vi "Add A File.vi"(5 "Size":u32, 7 "Parrent":string, 10 "Name":string, 11 "Map":T1) -> (3 "Map Out":T1)   [LabVIEW 2020]
uses:
  MAP_Structure.ctl
  Cluster_Item Data.ctl
  <vilib>/Utility/miscctls.llb/LVMapReplaceAction.ctl
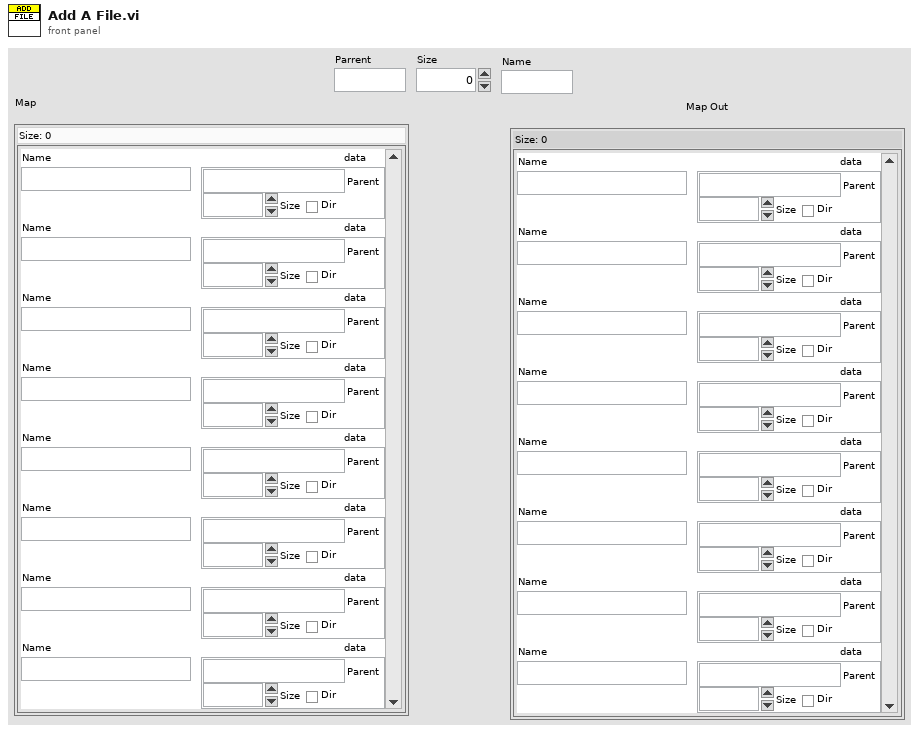
[diagram p1: front panel]
types:
  T1 = typedef "MAP_Structure.ctl" = map{string, T2}
  T2 = typedef "Cluster_Item Data.ctl" = cluster{"Parent":string, "Size":u32, "Dir":bool}
  T3 = typedef "LVMapReplaceAction.ctl" = enum32{"Modify Entry only if found", "Add or Modify Entry", "Delete Entry"}
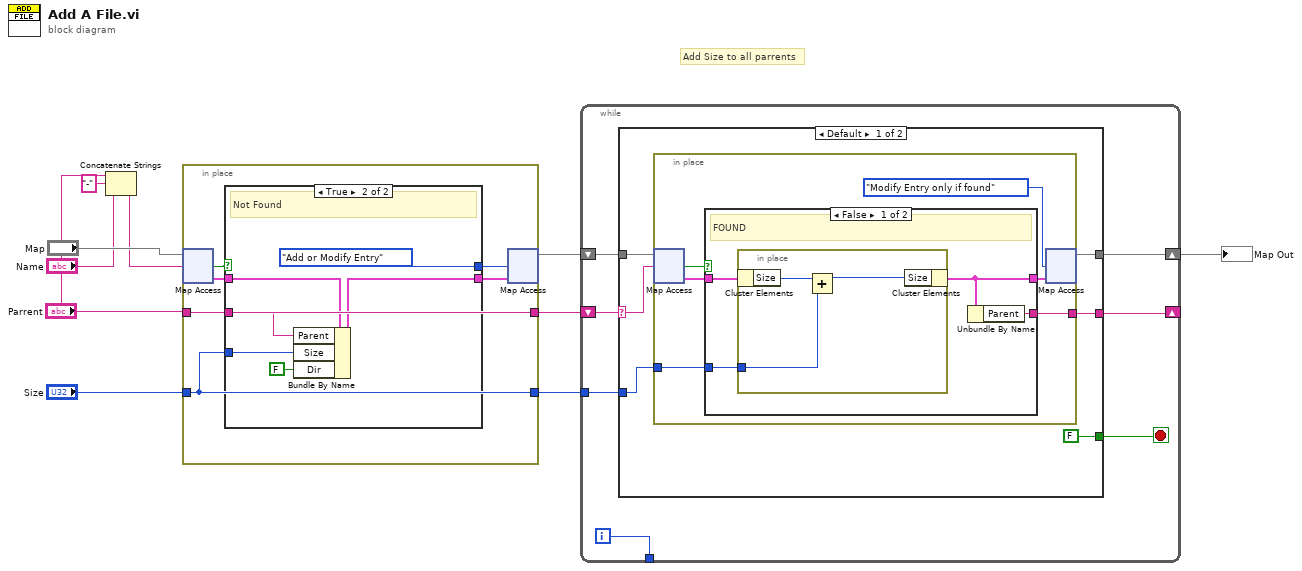
[diagram p0: block diagram]
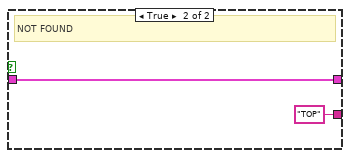
[diagram p2: hidden frame]
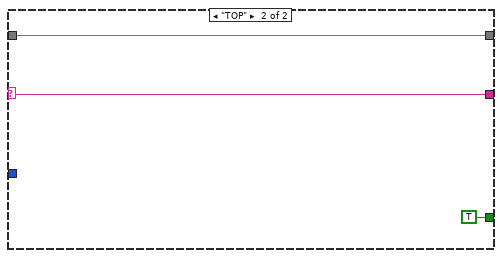
[diagram p3: hidden frame]
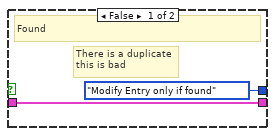
[diagram p4: hidden frame]
diagram:
  # "Add Size to all parrents"
  n1 = Concatenate Strings("Parrent", "-" ("string"), "Name") -> (w1:string)
  n2 = in-place {
    in-place-border: "Parrent" -> [w12]
    in-place-border: "Size" -> [w13]
    in-place-border: [w13] -> w6
    in-place-border: [w12] -> w5
    n3 = in-place-map #1("Map", w1) -> (w16:T2, w11:bool)  [unwired: 1 in]
    n4 = case shown="True" w11 {
      tunnel: w16 -> [w18 w24]
      tunnel: [w18 w23] -> w15
      tunnel: [LVMapReplaceAction."Modify Entry only if found" ("action") LVMapReplaceAction."Add or Modify Entry" ("action")] -> w14
      tunnel: w13 -> [_ w21]
      tunnel: w12 -> [_ w20]
      frame False {
        # "There is a duplicate\nthis is bad"
        # "Found"
      }
      frame True {
        # "Not Found"
        n5 = Bundle By Name(cluster=w24, "Parent"=w20, "Size"=w21, "Dir"=FALSE) -> (w23:T2)
      }
    }
    n6 = in-place-map #1(w15, w14) -> (w8:T1)  [unwired: 2 out]
  }
  n7 = while {
    shift-right: [w29] -> w7
    shift-left: w8 -> [w30]
    tunnel: w6 -> [w26]
    shift-right: [w27] -> _
    shift-left: w5 -> [w31]
    tunnel: [w25] -> _
    i -> [w25]
    stop <- w28 stop-if-true
    n8 = case shown="Default" w31 {
      selector: w31 -> [w34 w54]
      tunnel: w30 -> [w36 w55]
      tunnel: [w35 w55] -> w29
      tunnel: [FALSE TRUE] -> w28
      tunnel: [w33 w54] -> w27
      tunnel: w26 -> [w32 _]
      frame Default {
        n9 = in-place {
          in-place-border: [w41] -> w33
          in-place-border: w32 -> [w39]
          n10 = in-place-map #2(w36, w34) -> (w42:T2, w43:bool)  [unwired: 1 in]
          n11 = case shown="False" w43 {
            tunnel: w42 -> [w46 w52]
            tunnel: [w47 "TOP" ("Parent")] -> w41
            tunnel: [w45 w52] -> w40
            tunnel: w39 -> [w44 _]
            frame False {
              # "FOUND"
              n12 = in-place {
                in-place-border: w44 -> [w48]
                n13 = in-place-cluster #3(w46) -> ("Size"=w50:u32)
                n14 = Add(x=w50, y=w48) -> (x+y=w49:u32)
                n15 = in-place-cluster #3("Size"=w49) -> (w45:T2)
              }
              n16 = Unbundle By Name(w45) -> ("Parent"=w47:string)
            }
            frame True {
              # "NOT FOUND"
            }
          }
          n17 = in-place-map #2(w40, LVMapReplaceAction."Modify Entry only if found" ("action")) -> (w35:T1)  [unwired: 2 out]
        }
      }
      frame "TOP" {
      }
    }
  }
  "Map Out" <- w7
